vi "DataBroadcaster.vi"(0 "Data":string, 1 "Action":string) -> ()   [LabVIEW 2025]
uses:
  ServerGlobalVariables.vi
  ServerNetworkInterfaceGlobalVariables.vi
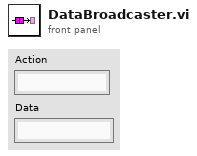
[diagram p1: front panel]
types:
  T1 = cluster{"Data":string, "Address":u32, "Port":u16}
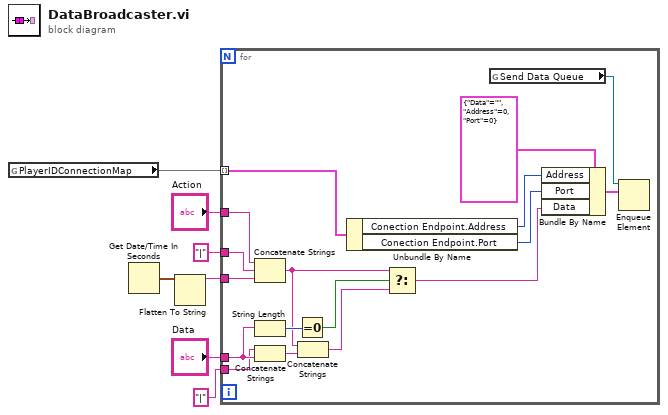
[diagram p0: block diagram]
diagram:
  n1 = global read "ServerGlobalVariables.vi" "PlayerIDConnectionMap"() -> (w7:map{u32, cluster{"Address":u32, "Port":u16}})
  n2 = Get Date/Time In Seconds() -> (seconds since 1Jan1904=w4:timestamp)
  n3 = Flatten To String(anything=w4) -> (data string=w3:string)  [unwired: 3 in, 2 out]
  n4 = for {
    tunnel: w7 -> [w24] mode=indexing
    tunnel: "Data" -> [w13]
    tunnel: "Action" -> [w14]
    tunnel: w3 -> [w18]
    tunnel: "|" ("Data") -> [w17]
    tunnel: "|" ("Data") -> [w12]
    n5 = Concatenate Strings(w14, w17, w18) -> (w8:string)
    n6 = String Length(string=w13) -> (length=w16:i32)
    n7 = Concatenate Strings(w12, w13) -> (w9:string)
    n8 = Equal To 0?(x=w16) -> (x = 0?=w15:bool)
    n9 = Concatenate Strings(w8, w9) -> (w10:string)
    n10 = Unbundle By Name(w24) -> ("Conection Endpoint.Address"=w23:u32, "Conection Endpoint.Port"=w22:u16)
    n11 = Select(t=w8, s=w15, f=w10) -> (s? t:f=w11:string)
    n12 = global read "ServerNetworkInterfaceGlobalVariables.vi" "Send Data Queue"() -> (w21:refnum<queue>)
    n13 = Bundle By Name(cluster=T1 {"Data"="", "Address"=0, "Port"=0}, "Address"=w23, "Port"=w22, "Data"=w11) -> (w19:T1)
    n14 = Enqueue Element(queue=w21, element=w19) -> ()  [unwired: 2 in, 3 out]
  }
